vi "ConfigureRobotProfile.vi"(0 "Selected Robot":i32) -> ()   [LabVIEW 2019]
doc: "Uses robot profile information to determine which sensors should be bypassed"
uses:
  robotprofile.vi
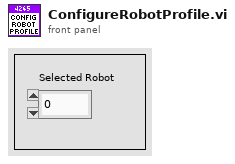
[diagram p1: front panel]
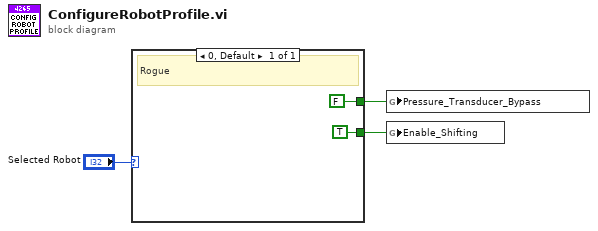
[diagram p0: block diagram]
diagram:
  n1 = case shown="0, Default" "Selected Robot" {
    tunnel: [FALSE ("Pressure_Transducer_Bypass")] -> w2
    tunnel: [TRUE ("Pressure_Transducer_Bypass")] -> w1
    frame 0, Default {
      # "Rogue"
    }
  }
  n2 = global write "robotprofile.vi" "Pressure_Transducer_Bypass"(w2) -> ()
  n3 = global write "robotprofile.vi" "Enable_Shifting"(w1) -> ()
